vi "Array Pile-up Correction [SGL].vi"(6 "Replace Inf by NaN (True)":bool=TRUE, 8 "Error In":errorcluster, 9 "Pixel Well Capacity":sgl, 11 "Image Pixels":sgl[](array[numeric])) -> (0 "Error Out":errorcluster, 1 "# Inf >> NaN Replacements":i32, 3 "Corrected Image Pixels":sgl[](array[numeric]))   [LabVIEW 2021, in "Arrays.lvlib"]
doc: "Computes the pile-up corrected values according to the following formula:\n\npucA[i] = -M*Ln(1-A[i]/M)\n\nwhere M is the <B>Pixel Well Capacity</b>, A[i] are the <B>Image Pixels</B> values and pucA[i] are the <B>Corrected Image Pixels</B>.\n\nIf <B>Replace Inf by NaN</B> is True, replaces +/-Inf returned values by NaN.\n\nAn error is returned if any of the <B>Image Pixels</B> is not positive or is larger than the <B>Pixel Well Capacity</B>."
uses:
  Arrays.lvlib
  461bb576-3a2d-4d03-91ca-083a3305c174.vi
  <vilib>/Utility/error.llb/Error Cluster From Error Code.vi
  <vilib>/ErrorRing/Error Ring.xnode
  Error/Error.lvlib
panel:
  # "see the AlliGator License on the block diagram (Ctrl+E or Window:Show Block Diagram)"
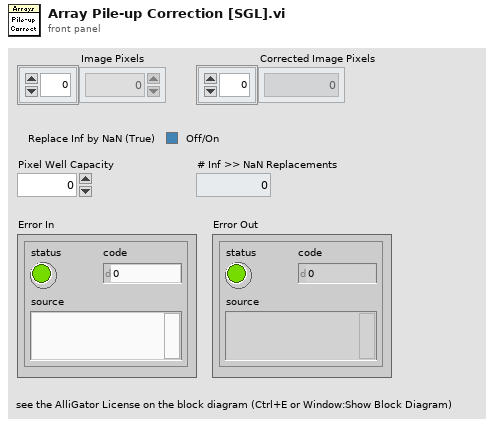
[diagram p1: front panel]
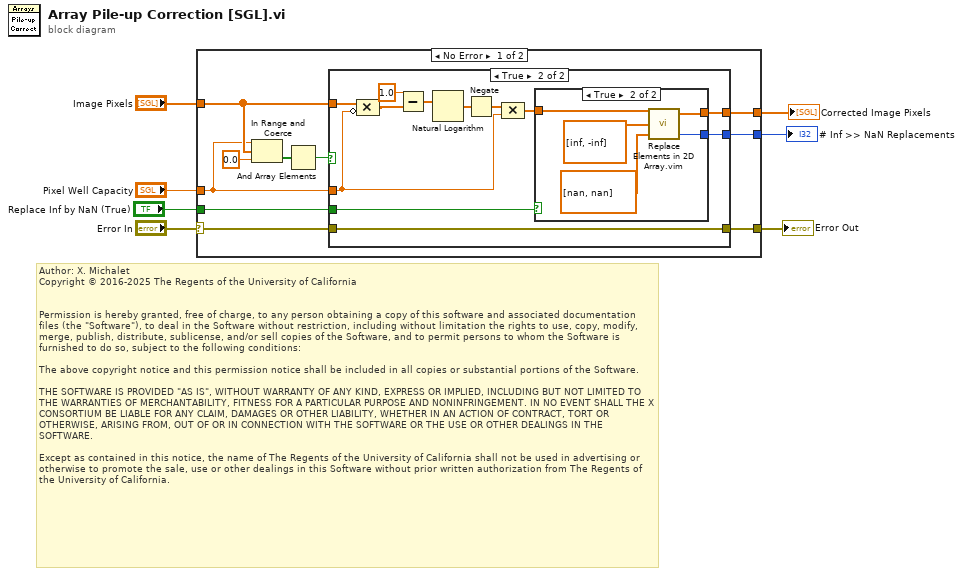
[diagram p0: block diagram]
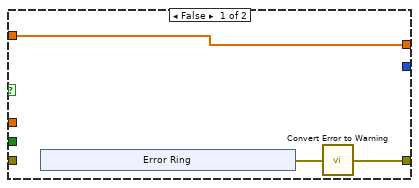
[diagram p2: hidden frame]
diagram:
  # "Author: X. Michalet\nCopyright © 2016-2025 The Regents of the University of California\n \n\nPermission is hereby granted, free of charge, to any person obtaining a copy of this software and associated documentation files (the \"Software\"), to deal in the Software without restriction, including without limitation the rights to use, copy, modify, merge, publish, distribute, sublicense, and/or sell copies of the Software, and to permit persons to whom the Software is furnished to do so, subject to the following conditions:\n\nThe above copyright notice and this permission notice shall be included in all copies or substantial portions of the Software.\n\nTHE SOFTWARE IS PROVIDED \"AS IS\", WITHOUT WARRANTY OF ANY KIND, EXPRESS OR IMPLIED, INCLUDING BUT NOT LIMITED TO THE WARRANTIES OF MERCHANTABILITY, FITNESS FOR A PARTICULAR PURPOSE AND NONINFRINGEMENT. IN NO EVENT SHALL THE X CONSORTIUM BE LIABLE FOR ANY CLAIM, DAMAGES OR OTHER LIABILITY, WHETHER IN AN ACTION OF CONTRACT, TORT OR OTHERWISE, ARISING FROM, OUT OF OR IN CONNECTION WITH THE SOFTWARE OR THE USE OR OTHER DEALINGS IN THE SOFTWARE.\n\nExcept as contained in this notice, the name of The Regents of the University of California shall not be used in advertising or otherwise to promote the sale, use or other dealings in this Software without prior written authorization from The Regents of the University of California."
  n1 = case shown="No Error" "Error In" {
    selector: "Error In" -> [w9 w43]
    tunnel: [w17 _] -> w7
    tunnel: "Pixel Well Capacity" -> [w13 _]
    tunnel: [w16 w44] -> w6
    tunnel: "Image Pixels" -> [w14 w44]
    tunnel: [w10 w43] -> w2
    tunnel: "Replace Inf by NaN (True)" -> [w8 _]
    frame No Error {
      n2 = In Range and Coerce(upper limit=w13, x=w14, lower limit=sgl 0.0) -> (In Range?=w12:bool[])  [unwired: 1 out]
      n3 = And Array Elements(Boolean array=w12) -> (logical AND=w11:bool)
      n4 = case shown="True" w11 {
        tunnel: [_ w36] -> w17
        tunnel: [w20 w35] -> w16
        tunnel: w14 -> [w20 w29]
        tunnel: w13 -> [_ w27]
        tunnel: [w18 w28] -> w10
        tunnel: w9 -> [_ w28]
        tunnel: w8 -> [_ w25]
        frame False {
          n5 = xnode "Error Ring"() -> ("error out"=w19:errorcluster)
          n6 = call "Convert Error to Warning.vi"("Error In"=w19) -> ("no Error Out"=w18:errorcluster)  [unwired: 8 in]
        }
        frame True {
          n7 = Compound Arithmetic op=MULTIPLY(w29, invert w27) -> (w32:sgl[])
          n8 = Subtract(x=sgl 1.0, y=w32) -> (x-y=w33:sgl[])
          n9 = Natural Logarithm(1:w33) -> (0:w30:sgl[])
          n10 = Negate(x=w30) -> (-x=w31:sgl[])
          n11 = Compound Arithmetic op=MULTIPLY(w31, w27) -> (w34:sgl[])
          n12 = case shown="True" w25 {
            tunnel: [_ w42] -> w36
            tunnel: [w37 w39] -> w35
            tunnel: w34 -> [w37 w38]
            frame False {
            }
            frame True {
              n13 = call "Replace Elements in 2D Array.vim"("Array"=w38, "Values to Replace"=sgl[] [inf, -inf], "Replacement Values"=sgl[] [nan, nan] ("Values to Replace")) -> ("Modified Array"=w39:sgl[], "# Replacements"=w42:i32)  [unwired: 5 in]
            }
          }
        }
      }
    }
    frame Error {
    }
  }
  "# Inf >> NaN Replacements" <- w7
  "Corrected Image Pixels" <- w6
  "Error Out" <- w2
